vi "2021_day6_task2.vi"() -> ()   [LabVIEW 2021]
panel:
  out "Arr to overflow":i32
  out "Iteration":i32
  out "# of fish(s)":i32
  in  "# of Iteration":i32=80
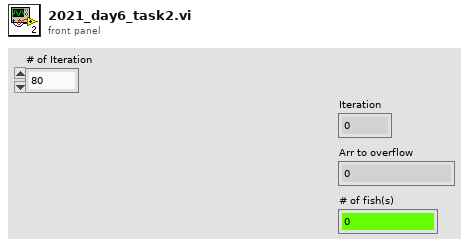
[diagram p1: front panel]
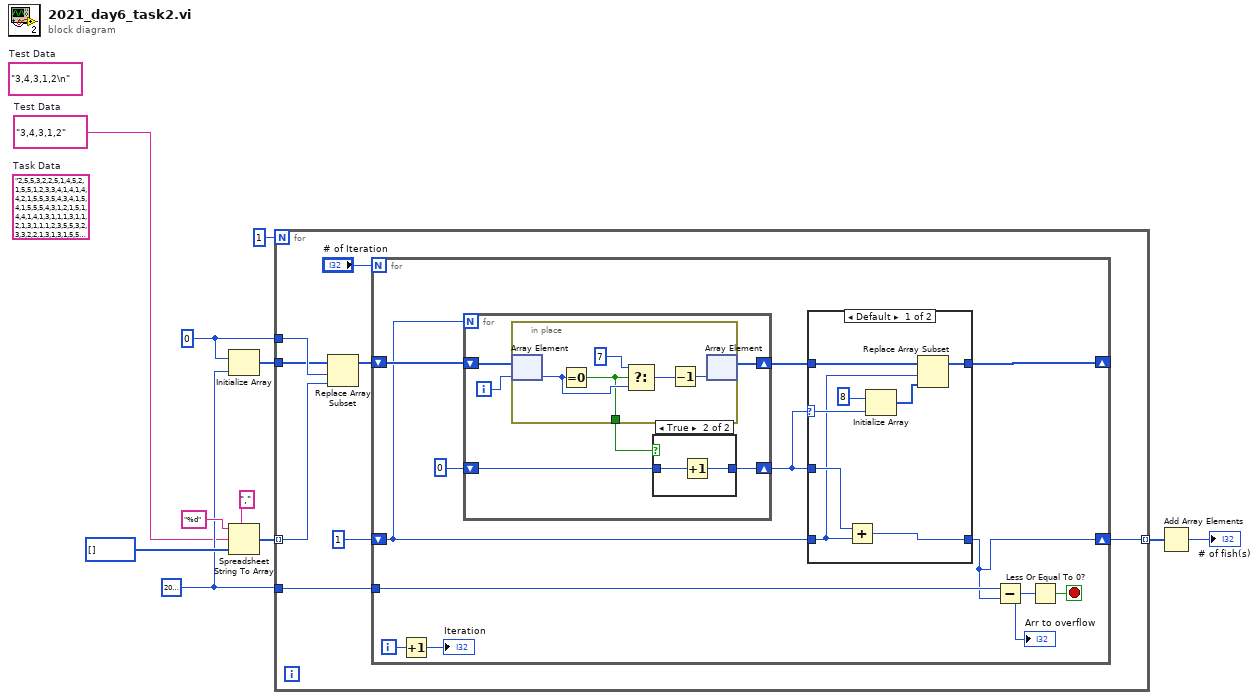
[diagram p0: block diagram]
diagram:
  w3 = i8 0
  (unwired) "3,4,3,1,2\n"  # Test Data
  w8 = 2000000000
  (unwired) "2,5,5,3,2,2,5,1,4,5,2,1,5,5,1,2,3,3,4,1,4,1,4,4,2,1,5,5,3,5,4,3,4,1,5,4,1,5,5,5,4,3,1,2,1,5,1,4,4,1,4,1,3,1,1,1,3,1,1,2,1,3,1,1,1,2,3,5,5,3,2,3,3,2,2,1,3,1,3,1,5,5,1,2,3,2,1,1,2,1,2,1,2,2,1,3,5,4,3,3,2,2,3,1,4,2,2,1,3,4,5,4,2,5,4,1,2,1,3,5,3,3,5,4,1,1,5,2,4,4,1,2,2,5,5,3,1,2,4,3,3,1,4,2,5,1,5,1,2,1,1,1,1,3,5,5,1,5,5,1,2,2,1,2,1,2,1,2,1,4,5,1,2,4,3,3,3,1,5,3,2,2,1,4,2,4,2,3,2,5,1,5,1,1,1,3,1,1,3,5,4,2,5,3,2,2,1,4,5,1,3,2,5,1,2,1,4,1,5,5,1,2,2,1,2,4,5,3,3,1,4,4,3,1,4,2,4,4,3,4,1,4,5,3,1,4,2,2,3,4,4,4,1,4,3,1,3,4,5,1,5,4,4,4,5,5,5,2,1,3,4,3,2,5,3,1,3,2,2,3,1,4,5,3,5,5,3,2,3,1,2,5,2,1,3,1,1,1,5,1"  # Task Data
  w6 = "3,4,3,1,2"  # Test Data
  n1 = Initialize Array(w3, w8) -> (w2:i8[])
  n2 = Spreadsheet String To Array(delimiter (Tab)=",", format string="%d", spreadsheet string=w6, array type (2D Dbl)=i8[] []) -> (array=w7:i8[])
  n3 = for {
    N: 1 -> [_]
    tunnel: w8 -> [w18]
    tunnel: w7 -> [w15] mode=indexing
    tunnel: [w16] -> w5 mode=indexing
    tunnel: w3 -> [w14]
    tunnel: w2 -> [w13]
    n4 = Replace Array Subset(array=w13, new element=w15, index=w14) -> (w17:i8[])
    n5 = for {
      N: "# of Iteration" -> [_]
      shift-right: [w25] -> _
      shift-left: w17 -> [w27]
      shift-right: [w23] -> w16
      shift-left: 1 -> [w22]
      tunnel: w18 -> [w29]
      i -> [w30]
      stop <- w28 stop-if-true
      n6 = Increment(x=w30) -> (x+1=→"Iteration":i32)
      n7 = for {
        N: w22 -> [_]
        shift-right: [w45] -> w31
        shift-left: w27 -> [w47]
        shift-right: [w43] -> w24
        shift-left: 0 -> [w44]
        i -> [w46]
        n8 = in-place {
          in-place-border: [w52] -> w42
          n9 = in-place-array #1(w47, w46) -> (w53:i8)
          n10 = Equal To 0?(x=w53) -> (x = 0?=w52:bool)
          n11 = Select(t=i8 7, s=w52, f=w53) -> (s? t:f=w54:i8)
          n12 = Decrement(x=w54) -> (x-1=w51:i8)
          n13 = in-place-array #1(w51) -> (w45:i8[])  [unwired: 1 out]
        }
        n14 = case shown="True" w42 {
          tunnel: w44 -> [w48 w50]
          tunnel: [w48 w49] -> w43
          frame False {
          }
          frame True {
            n15 = Increment(x=w50) -> (x+1=w49:i32)
          }
        }
      }
      n16 = case shown="Default" w24 {
        selector: w24 -> [w36 _]
        tunnel: w31 -> [w39 w41]
        tunnel: [w38 w41] -> w25
        tunnel: w24 -> [w34 _]
        tunnel: w22 -> [w32 w40]
        tunnel: [w33 w40] -> w23
        frame Default {
          n17 = Add(x=w34, y=w32) -> (x+y=w33:i32)
          n18 = Initialize Array(i8 8, w36) -> (w37:i8[])
          n19 = Replace Array Subset(array=w39, new element=w37, index=w32) -> (w38:i8[])
        }
        frame 0 {
        }
      }
      n20 = Subtract(x=w29, y=w23) -> (x-y=w21:i32)
      "Arr to overflow" <- w21
      n21 = Less Or Equal To 0?(x=w21) -> (x <= 0?=w28:bool)
    }
  }
  n22 = Add Array Elements(numeric array=w5) -> (sum=→"# of fish(s)":i32)
